vi "Clear Specified Error.vi"(0 "error in (no error)":errorcluster, 1 "Code to Clear (0)":i32) -> (2 "error out":errorcluster)   [LabVIEW 2023]
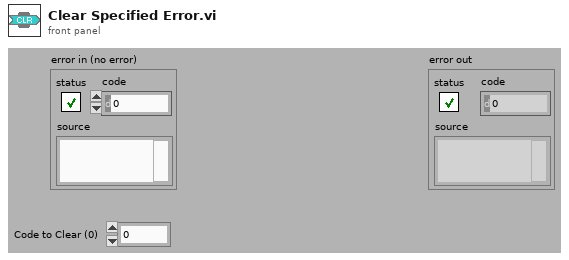
[diagram p1: front panel]
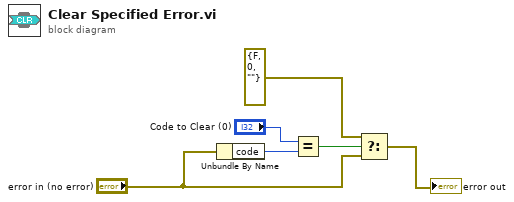
[diagram p0: block diagram]
diagram:
  n1 = Unbundle By Name("error in (no error)") -> ("code"=w6:i32)
  n2 = Equal?(x="Code to Clear (0)", y=w6) -> (x = y?=w4:bool)
  n3 = Select(t=errorcluster {"status"=FALSE, "code"=0, "source"=""}, s=w4, f="error in (no error)") -> (s? t:f=→"error out":errorcluster)
